vi "GUI FOFB Configuration Window.vi"(9 "username":string, 10 "password":string, 11 "FOFB-Controller IP Address in":string="10.0.5.31") -> (3 "Cancelled?":bool)   [LabVIEW 2011, in "User Interface Window VIs.lvlib"]
doc: "Fast Orbit Feedback (FOFB) graphical user interface."
uses:
  User Interface Window VIs.lvlib
  Types Definitions/Type BPM or PS Selector.ctl
  Types Definitions/Type FOFB Parameters.ctl
  Types Definitions/Type Network Configuration.ctl
  Types Definitions/Type FA Configuration.ctl
  Types Definitions/Type Response Matrix Measurement Configuration.ctl
  Types Definitions/Type Correction Algorithm Configuration.ctl
  Types Definitions/Type Acquisition Network Configuration.ctl
  Types Definitions/Type Actuation Network Configuration.ctl
  Types Definitions/Type FOFB GUI.ctl
  Types Definitions/Type Configuration Loop Mode.ctl
  Types Definitions/Type Configuration Data (GUI to Controller).ctl
  Types Definitions/Type Monitoring Data.ctl
  Types Definitions/Type Diagnostics Data.ctl
  Types Definitions/Type CPU Loads Array.ctl
  Types Definitions/Type CPU Loads.ctl
  Types Definitions/Type Diagnostics Sample.ctl
  Types Definitions/Type Monitoring Sample.ctl
  User Interface VIs.lvlib
  Type Definitions.lvlib
  XML VIs.lvlib
panel:
  in  "FOFB GUI In":T1
  out "FOFB Parameters Out":T2
  in  "FOFB Parameters In":T2
  in  "Refresh Button":bool
  out "Response Matrix List":string[](array[string]) caption="Lista de Matrizes Resposta"
  in  "Response Matrix":string caption="Matriz Resposta Escolhida"
  in  "PS Group ALV":bool
  in  "PS Group ACV":bool
  in  "PS Group ACH":bool
  in  "BPM Selector Vertical":bool
  in  "BPM Selector Horizontal":bool
  in  "PS Graph Selector ALV":T9[](array[typedef]) caption="Grupo ALV"
  in  "PS Graph Selector Vertical":T9[](array[typedef]) caption="Grupo ACV"
  in  "PS Graph Selector Horizontal":T9[](array[typedef]) caption="Grupo ACH"
  in  "BPM Graph Selector Vertical":T9[](array[typedef]) caption="BPMs Verticais"
  in  "BPM Graph Selector Horizontal":T9[](array[typedef]) caption="BPMs Horizontais"
  in  "Cancel Button":bool
  in  "OK Button":bool
  in  "BPM Graph Selector":T9[](array[typedef]) caption="BPMs"
  in  "Vertical (%)":dbl
  in  "Horizontal (%)":dbl
  # "Todos/Nenhum"
  # "Todos/Nenhum"
  # "Todos/Nenhum"
  # "Todos/Nenhum"
  # "Todos/Nenhum"
  # "Fator de correção"
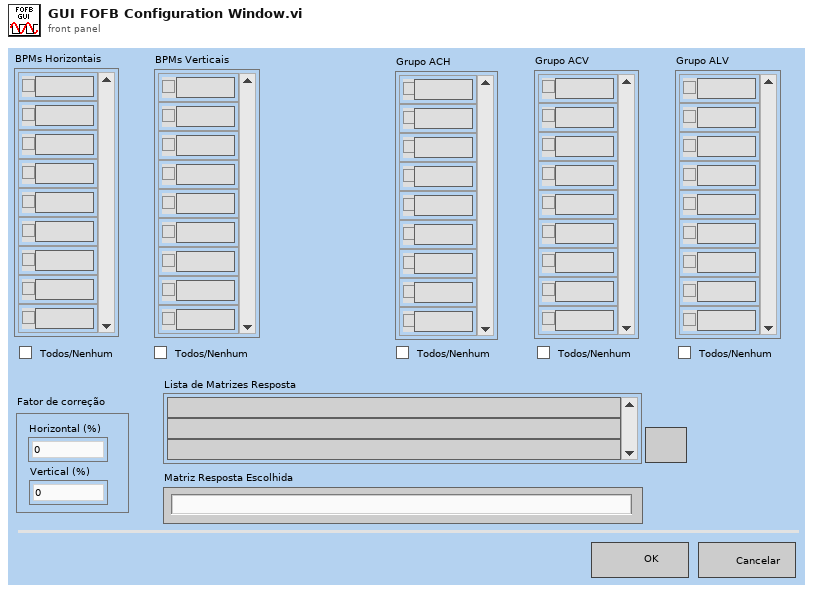
[diagram p1: front panel]
types:
  T1 = typedef "Type Definitions.lvlib/Type FOFB GUI.ctl" = cluster{"Response Matrix List Folder Notifier":refnum<notifier>, "Send Reference Orbit Notifier":refnum<notifier>, "FOFB Parameters Notifier":refnum<notifier>, "Configuration Loop Mode Notifier":refnum<notifier>, "Stop VIs Notifier":refnum<notifier>, "GUI Configuration Notifier":refnum<notifier>, "Monitoring Data Notifier":refnum<queue>, "Performance Monitoring Data Notifier":refnum<queue>, "BPM / PS Monitoring Data Notifiers":refnum<queue>[], "Load Orbit Notifier":refnum<notifier>, "RMS Monitoring Data Queue":refnum<queue>, "GUI-Controller Connected Queue":refnum<queue>}
  T2 = typedef "Type Definitions.lvlib/Type FOFB Parameters.ctl" = cluster{"Network":T3, "Fast Acquisition":T4, "Response Matrix Measurement":T5, "Correction Algorithm":T6, "Acquisition Network":T7, "Actuation Network":T8}
  T3 = typedef "Type Definitions.lvlib/Type Network Configuration.ctl" = cluster{"FOFB Controller IP":string, "LNLS Control Network IP":string, "LNLS Control Network Power Supplies TCP Port":u16, "LNLS Control Network FOFB Configuration TCP Port":u16, "Data Server TCP Port":u16, "Monitoring Data TCP Port":u16, "Configuration GUI TCP Port":u16, "TCP Listening Timeout":i32}
  T4 = typedef "Type Definitions.lvlib/Type FA Configuration.ctl" = cluster{"Acquisition Period":u32, "Data Buffer Size":u32, "Monitoring Period":u32}
  T5 = typedef "Type Definitions.lvlib/Type Response Matrix Measurement Configuration.ctl" = cluster{"Step Amplitude":dbl, "Time Between Steps":u32, "Step Duration":u32, "Number of Averages":u32}
  T6 = typedef "Type Definitions.lvlib/Type Correction Algorithm Configuration.ctl" = cluster{"Correction Period":u32, "Reference Orbit Path":path, "Response Matrix Path":path, "Correction Matrix Path":path, "Horizontal Correction Factor":dbl, "Vertical Correction Factor":dbl, "Beam Current FOFB Threshold":dbl, "Decouple H-V":bool, "Use Additional BPM LPF":bool, "BPM LPF Cutoff":dbl}
  T7 = typedef "Type Definitions.lvlib/Type Acquisition Network Configuration.ctl" = cluster{"Chassis Name":string, "Variables":cluster{"Variable Name":string, "Matrix Order":u32, "Location":dbl, "Plane":enum8{"H", "V"}, "On Correction":bool}[]}[]
  T8 = typedef "Type Definitions.lvlib/Type Actuation Network Configuration.ctl" = cluster{"Chassis Name":string, "Variables":cluster{"Variable Name":string, "Matrix Order":u32, "RMM Step Factor":dbl, "Plane":enum8{"H", "V"}, "On Correction":bool, "Kc":dbl, "Ti":dbl, "Td":dbl}[]}[]
  T9 = typedef "Type Definitions.lvlib/Type BPM or PS Selector.ctl" = cluster{"Name":string, "Active":bool}
  T10 = typedef "Type Definitions.lvlib/Type Configuration Loop Mode.ctl" = enum8{"Operation Mode", "Request FOFB Parameters", "Send New FOFB Parameters", "Send Reference Orbit", "Request Response Matrix List Folder"}
  T11 = typedef "Type Definitions.lvlib/Type PS Parameters.ctl" = cluster{"RMM Step Factor":dbl, "Plane":enum8{"H", "V"}, "On Correction":bool}
  T12 = typedef "Type Definitions.lvlib/Type BPM Parameters.ctl" = cluster{"Location":dbl, "Plane":enum8{"H", "V"}, "On Correction":bool}
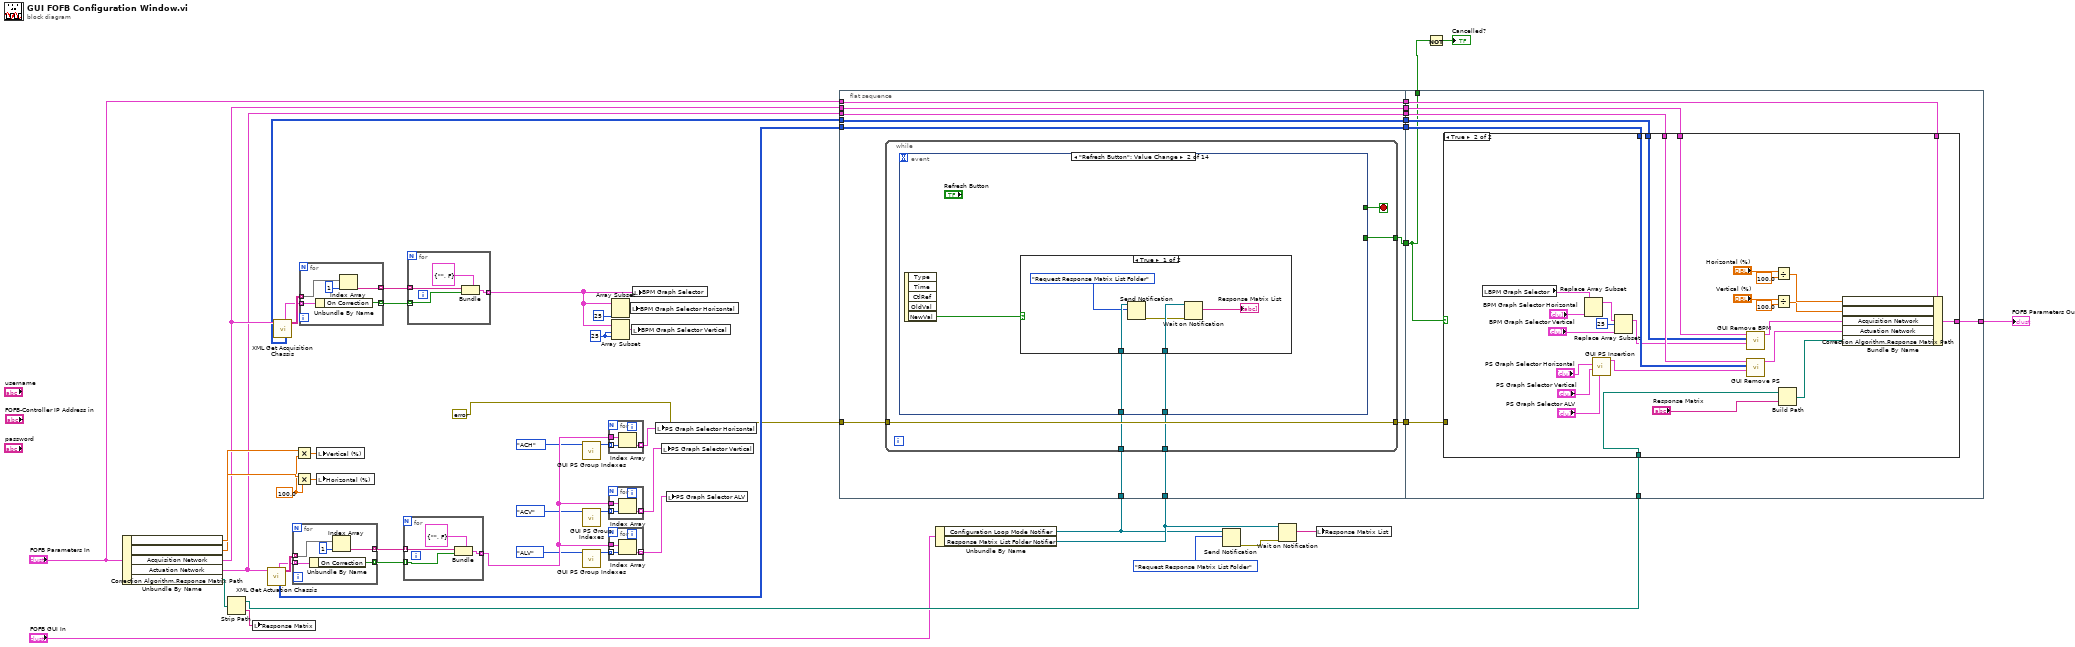
[diagram p0: block diagram]
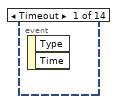
[diagram p2: hidden frame]
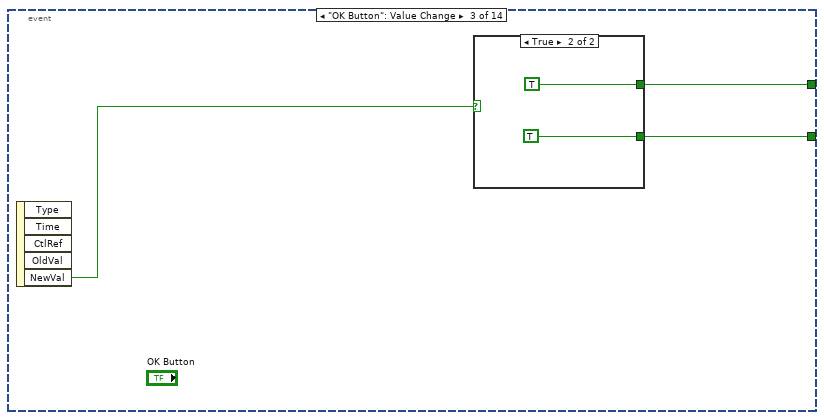
[diagram p4: hidden frame]
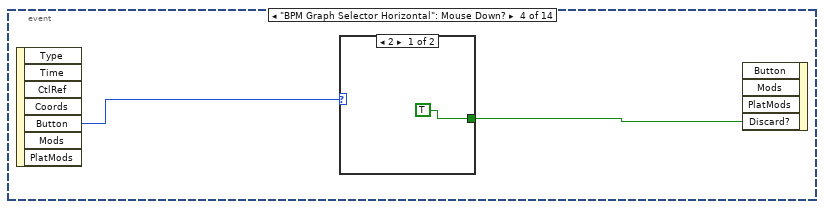
[diagram p6: hidden frame]
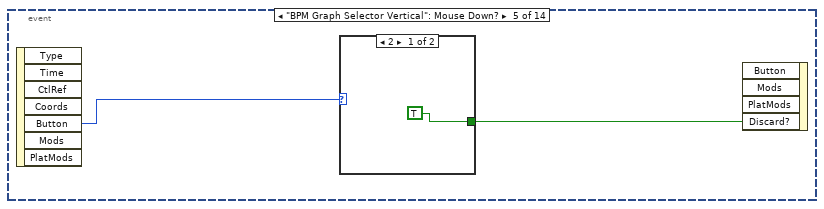
[diagram p8: hidden frame]
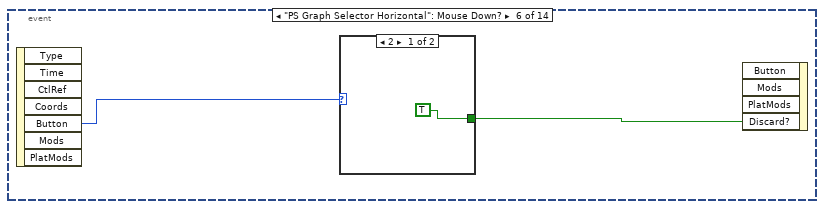
[diagram p10: hidden frame]
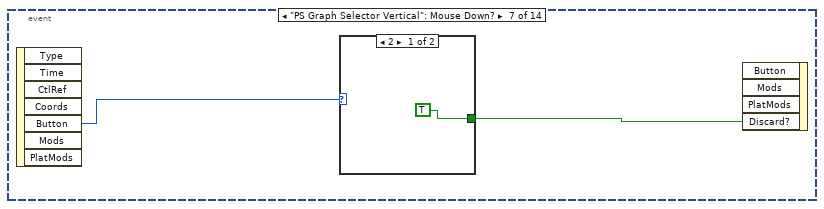
[diagram p12: hidden frame]
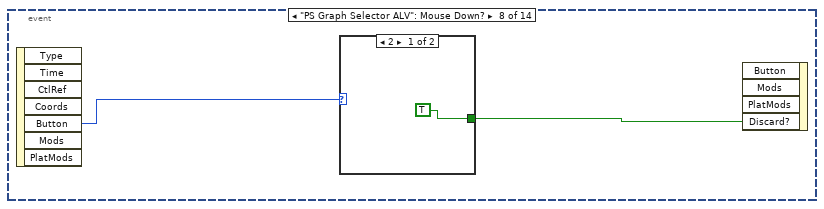
[diagram p14: hidden frame]
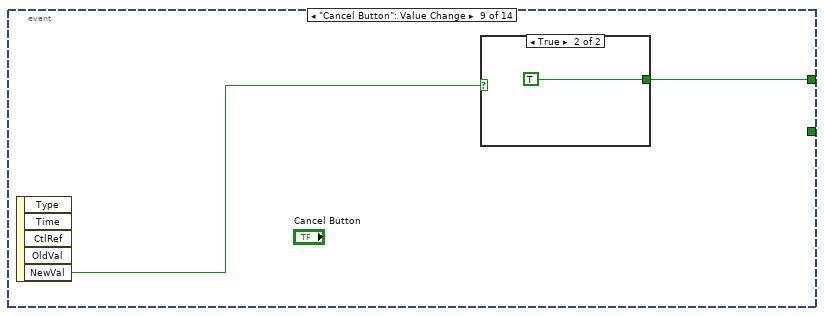
[diagram p16: hidden frame]
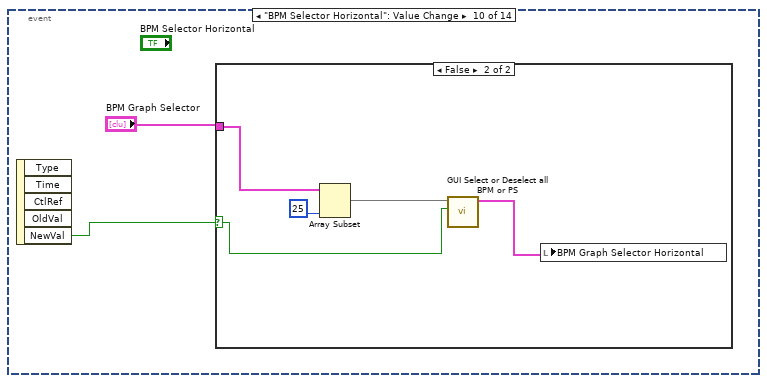
[diagram p18: hidden frame]
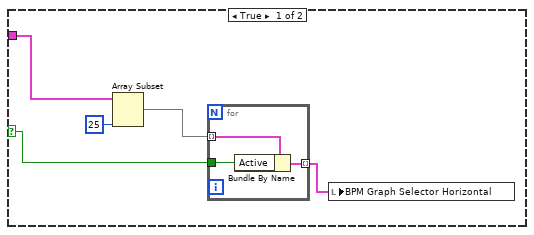
[diagram p19: hidden frame]
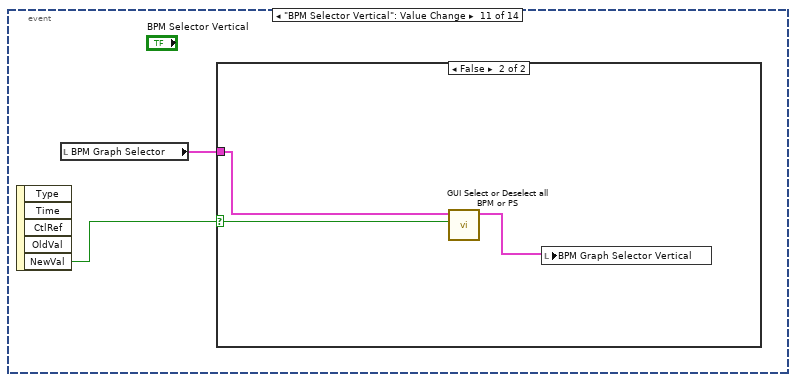
[diagram p20: hidden frame]
diagram:
  w17 = 25 ("index")
  w40 = 100.0 ("y")
  n1 = Unbundle By Name("FOFB Parameters In") -> ("Correction Algorithm.Horizontal Correction Factor"=w43:dbl, "Correction Algorithm.Vertical Correction Factor"=w42:dbl, "Acquisition Network"=w39:T7, "Actuation Network"=w38:T8, "Correction Algorithm.Response Matrix Path"=w31:path)
  n2 = Strip Path(path=w31) -> (stripped path=w30:path, name=w32:string)
  n3 = local write "Response Matrix"(w32) -> ()
  n4 = call "XML Get Actuation Chassis.vi"("Actuation Network"=w38) -> ("Actuation Variable Names"=w49:string[][], "Inverse PS Matrix Mapping"=w36:u32[][], "PS Parameters"=w48:T11[])  [unwired: 3 in, 5 out]
  n5 = call "XML Get Acquisition Chassis.vi"("Acquisition Network"=w39) -> ("Acquisition Variable Names"=w52:string[][], "Inverse BPM Matrix Mapping"=w37:u32[][], "BPM Parameters"=w47:T12[])  [unwired: 4 in, 4 out]
  n6 = for {
    tunnel: w49 -> [w57] mode=indexing
    tunnel: [w56] -> w46 mode=indexing
    tunnel: w48 -> [w55] mode=indexing
    tunnel: [w54] -> w45 mode=indexing
    n7 = Unbundle By Name(w55) -> ("On Correction"=w54:bool)
    n8 = Index Array(array=w57, index=1) -> (element=w56:string)
  }
  n9 = Multiply(x=w42, y=w40) -> (x*y=w41:dbl)
  n10 = Multiply(x=w43, y=w40) -> (x*y=w44:dbl)
  n11 = for {
    tunnel: w52 -> [w62] mode=indexing
    tunnel: [w61] -> w50 mode=indexing
    tunnel: w47 -> [w60] mode=indexing
    tunnel: [w59] -> w51 mode=indexing
    n12 = Unbundle By Name(w60) -> ("On Correction"=w59:bool)
    n13 = Index Array(array=w62, index=1) -> (element=w61:string)
  }
  n14 = local write "Vertical (%)"(w41) -> ()
  n15 = local write "Horizontal (%)"(w44) -> ()
  n16 = for {
    tunnel: [w66] -> w33 mode=indexing
    tunnel: w45 -> [w64] mode=indexing
    tunnel: w46 -> [w65] mode=indexing
    n17 = Bundle(cluster=T9 {"Name"="", "Active"=FALSE} ("BPM or PS Selection"), "Name"=w65, "Active"=w64) -> (w66:T9)
  }
  n18 = for {
    tunnel: [w70] -> w34 mode=indexing
    tunnel: w51 -> [w68] mode=indexing
    tunnel: w50 -> [w69] mode=indexing
    n19 = Bundle(cluster=T9 {"Name"="", "Active"=FALSE} ("BPM or PS Selection"), "Name"=w69, "Active"=w68) -> (w70:T9)
  }
  n20 = call "GUI PS Group Indexes.vi"("PS Group"=enum16{"ACH", "ACV", "ALV"}."ACH") -> ("Indexes"=w13:i32[])  [unwired: 10 in]
  n21 = call "GUI PS Group Indexes.vi"("PS Group"=enum16{"ACH", "ACV", "ALV"}."ACV") -> ("Indexes"=w11:i32[])  [unwired: 10 in]
  n22 = call "GUI PS Group Indexes.vi"("PS Group"=enum16{"ACH", "ACV", "ALV"}."ALV") -> ("Indexes"=w10:i32[])  [unwired: 10 in]
  n23 = for {
    tunnel: w33 -> [w74]
    tunnel: [w73] -> w15 mode=indexing
    tunnel: w13 -> [w72] mode=indexing
    n24 = Index Array(array=w74, index=w72) -> (element=w73:T9)
  }
  n25 = for {
    tunnel: w33 -> [w77]
    tunnel: [w76] -> w12 mode=indexing
    tunnel: w11 -> [w75] mode=indexing
    n26 = Index Array(array=w77, index=w75) -> (element=w76:T9)
  }
  n27 = for {
    tunnel: w33 -> [w80]
    tunnel: [w79] -> w14 mode=indexing
    tunnel: w10 -> [w78] mode=indexing
    n28 = Index Array(array=w80, index=w78) -> (element=w79:T9)
  }
  n29 = Array Subset(array=w34, length=25) -> (w18:T9[])  [unwired: 1 in]
  n30 = Array Subset(array=w34, index=w17, length=w17) -> (w19:T9[])
  n31 = local write "BPM Graph Selector Horizontal"(w18) -> ()
  n32 = local write "BPM Graph Selector Vertical"(w19) -> ()
  n33 = local write "BPM Graph Selector"(w34) -> ()
  n34 = local write "PS Graph Selector Horizontal"(w15) -> ()
  n35 = local write "PS Graph Selector Vertical"(w12) -> ()
  n36 = local write "PS Graph Selector ALV"(w14) -> ()
  n37 = flat-sequence {
    tunnel: errorcluster {"status"=FALSE, "code"=0, "source"=""} ("error in (no error)") -> [w83]
    tunnel: "FOFB Parameters In" -> [w89]
    tunnel: w39 -> [w88]
    tunnel: w38 -> [w87]
    tunnel: w37 -> [w86]
    tunnel: w36 -> [w85]
    tunnel: [w90] -> w26
    tunnel: [w89] -> w25
    tunnel: [w88] -> w24
    tunnel: [w87] -> w23
    tunnel: [w86] -> w22
    tunnel: [w85] -> w21
    tunnel: [w84] -> w20
    tunnel: w2 -> [w82]
    tunnel: w3 -> [w81]
    tunnel: w26 -> [w187]
    tunnel: w25 -> [w194]
    tunnel: w24 -> [w193]
    tunnel: w23 -> [w192]
    tunnel: w22 -> [w191]
    tunnel: w21 -> [w190]
    tunnel: [w187] -> w35
    tunnel: w30 -> [w189]
    tunnel: w20 -> [w188]
    tunnel: [w186] -> w27
    frame #0 {
      n38 = while {
        tunnel: w83 -> [w95]
        tunnel: [w95] -> w84
        tunnel: [w93] -> w90
        tunnel: w82 -> [w92]
        tunnel: w81 -> [w91]
        stop <- w94 stop-if-true
        n39 = event shown="[1] \"Refresh Button\": Value Change" {
          selector: _ -> [_ _ _ _ _ _ _ _ _ _ _ _ _ _]
          dyn-events: _ -> [_ _ _ _ _ _ _ _ _ _ _ _ _ _]
          timeout: _ -> [_ _ _ _ _ _ _ _ _ _ _ _ _ _]
          tunnel: [_ _ w106 _ _ _ _ _ w125 _ _ _ _ _] -> w94
          tunnel: [_ _ w105 _ _ _ _ _ _ _ _ _ _ _] -> w93
          tunnel: w92 -> [_ w97 _ _ _ _ _ _ _ _ _ _ _ _]
          tunnel: w91 -> [_ w96 _ _ _ _ _ _ _ _ _ _ _ _]
          event Timeout {
            n40 = event-data() -> ()  [unwired: 1 in, 2 out]
          }
          event "Refresh Button": Value Change {
            n41 = event-data() -> ("NewVal"=w98:bool)  [unwired: 1 in, 4 out]
            n42 = case shown="True" w98 {
              tunnel: w97 -> [w103 _]
              tunnel: w96 -> [w102 _]
              frame True {
                n43 = Send Notification(notification=Type_Configuration_Loop_Mode."Request Response Matrix List Folder", notifier=w103) -> (error out=w100:errorcluster)  [unwired: 1 in, 1 out]
                n44 = Wait on Notification(notifier=w102, error in (no error)=w100) -> (notification=→"Response Matrix List":string[])  [unwired: 2 in, 3 out]
              }
              frame False {
              }
            }
          }
          event "OK Button": Value Change {
            n45 = event-data() -> ("NewVal"=w104:bool)  [unwired: 1 in, 4 out]
            n46 = case shown="True" w104 {
              tunnel: [_ TRUE] -> w106
              tunnel: [_ TRUE] -> w105
              frame False {
              }
              frame True {
              }
            }
          }
          event "BPM Graph Selector Horizontal": Mouse Down? {
            n47 = event-data() -> ("Button"=w110:u16)  [unwired: 1 in, 6 out]
            n48 = case shown="2" w110 {
              tunnel: [TRUE ("Discard?") _] -> w109
              frame 2 {
              }
              frame 1, Default {
              }
            }
            n49 = event-data("Discard?"=w109) -> ()  [unwired: 4 in, 1 out]
          }
          event "BPM Graph Selector Vertical": Mouse Down? {
            n50 = event-data() -> ("Button"=w113:u16)  [unwired: 1 in, 6 out]
            n51 = case shown="2" w113 {
              tunnel: [TRUE ("Discard?") _] -> w112
              frame 2 {
              }
              frame 1, Default {
              }
            }
            n52 = event-data("Discard?"=w112) -> ()  [unwired: 4 in, 1 out]
          }
          event "PS Graph Selector Horizontal": Mouse Down? {
            n53 = event-data() -> ("Button"=w116:u16)  [unwired: 1 in, 6 out]
            n54 = case shown="2" w116 {
              tunnel: [TRUE ("Discard?") _] -> w115
              frame 2 {
              }
              frame 1, Default {
              }
            }
            n55 = event-data("Discard?"=w115) -> ()  [unwired: 4 in, 1 out]
          }
          event "PS Graph Selector Vertical": Mouse Down? {
            n56 = event-data() -> ("Button"=w119:u16)  [unwired: 1 in, 6 out]
            n57 = case shown="2" w119 {
              tunnel: [TRUE ("Discard?") _] -> w118
              frame 2 {
              }
              frame 1, Default {
              }
            }
            n58 = event-data("Discard?"=w118) -> ()  [unwired: 4 in, 1 out]
          }
          event "PS Graph Selector ALV": Mouse Down? {
            n59 = event-data() -> ("Button"=w122:u16)  [unwired: 1 in, 6 out]
            n60 = case shown="2" w122 {
              tunnel: [TRUE ("Discard?") _] -> w121
              frame 2 {
              }
              frame 1, Default {
              }
            }
            n61 = event-data("Discard?"=w121) -> ()  [unwired: 4 in, 1 out]
          }
          event "Cancel Button": Value Change {
            n62 = event-data() -> ("NewVal"=w124:bool)  [unwired: 1 in, 4 out]
            n63 = case shown="True" w124 {
              tunnel: [_ TRUE] -> w125
              frame False {
              }
              frame True {
              }
            }
          }
          event "BPM Selector Horizontal": Value Change {
            n64 = event-data() -> ("NewVal"=w128:bool)  [unwired: 1 in, 4 out]
            n65 = case shown="False" w128 {
              selector: w128 -> [w131 w137]
              tunnel: "BPM Graph Selector" -> [w129 w140]
              frame True {
                n66 = Array Subset(array=w129, length=25) -> (w132:T9[])  [unwired: 1 in]
                n67 = for {
                  tunnel: w132 -> [w135] mode=indexing
                  tunnel: [w136] -> w130 mode=indexing
                  tunnel: w131 -> [w134]
                  n68 = Bundle By Name(cluster=w135, "Active"=w134) -> (w136:T9)
                }
                n69 = local write "BPM Graph Selector Horizontal"(w130) -> ()
              }
              frame False {
                n70 = Array Subset(array=w140, length=25) -> (w139:T9[])  [unwired: 1 in]
                n71 = call "GUI Select or Deselect all BPM or PS.vi"("Boolean Value"=w137, "Variable Selector In"=w139) -> ("Variable Selector Out"=w138:T9[])  [unwired: 8 in, 1 out]
                n72 = local write "BPM Graph Selector Horizontal"(w138) -> ()
              }
            }
          }
          event "BPM Selector Vertical": Value Change {
            n73 = event-data() -> ("NewVal"=w143:bool)  [unwired: 1 in, 4 out]
            n74 = local read "BPM Graph Selector"() -> (w142:T9[])
            n75 = case shown="False" w143 {
              selector: w143 -> [w146 w151]
              tunnel: w142 -> [w144 w152]
              frame True {
                n76 = for {
                  tunnel: w144 -> [w148] mode=indexing
                  tunnel: [w149] -> w145 mode=indexing
                  tunnel: w146 -> [w147]
                  n77 = Bundle By Name(cluster=w148, "Active"=w147) -> (w149:T9)
                }
                n78 = local write "BPM Graph Selector Vertical"(w145) -> ()
              }
              frame False {
                n79 = call "GUI Select or Deselect all BPM or PS.vi"("Boolean Value"=w151, "Variable Selector In"=w152) -> ("Variable Selector Out"=w150:T9[])  [unwired: 8 in, 1 out]
                n80 = local write "BPM Graph Selector Vertical"(w150) -> ()
              }
            }
          }
          event "PS Group ACH": Value Change {
            n81 = event-data() -> ("NewVal"=w154:bool)  [unwired: 1 in, 4 out]
            n82 = local read "PS Graph Selector Horizontal"() -> (w153:T9[])
            n83 = case shown="True" w154 {
              selector: w154 -> [w155 w160]
              tunnel: w153 -> [w157 w158]
              frame True {
                n84 = call "GUI Select or Deselect all BPM or PS.vi"("Boolean Value"=w155, "Variable Selector In"=w157) -> ("Variable Selector Out"=w156:T9[])  [unwired: 8 in, 1 out]
                n85 = local write "PS Graph Selector Horizontal"(w156) -> ()
              }
              frame False {
                n86 = for {
                  tunnel: w158 -> [w163] mode=indexing
                  tunnel: [w162] -> w159 mode=indexing
                  tunnel: w160 -> [w161]
                  n87 = Bundle By Name(cluster=w163, "Active"=w161) -> (w162:T9)
                }
                n88 = local write "PS Graph Selector Horizontal"(w159) -> ()
              }
            }
          }
          event "PS Group ACV": Value Change {
            n89 = local read "PS Graph Selector Vertical"() -> (w164:T9[])
            n90 = event-data() -> ("NewVal"=w165:bool)  [unwired: 1 in, 4 out]
            n91 = case shown="True" w165 {
              selector: w165 -> [w166 w171]
              tunnel: w164 -> [w168 w169]
              frame True {
                n92 = call "GUI Select or Deselect all BPM or PS.vi"("Boolean Value"=w166, "Variable Selector In"=w168) -> ("Variable Selector Out"=w167:T9[])  [unwired: 8 in, 1 out]
                n93 = local write "PS Graph Selector Vertical"(w167) -> ()
              }
              frame False {
                n94 = for {
                  tunnel: w169 -> [w174] mode=indexing
                  tunnel: [w173] -> w170 mode=indexing
                  tunnel: w171 -> [w172]
                  n95 = Bundle By Name(cluster=w174, "Active"=w172) -> (w173:T9)
                }
                n96 = local write "PS Graph Selector Vertical"(w170) -> ()
              }
            }
          }
          event "PS Group ALV": Value Change {
            n97 = event-data() -> ("NewVal"=w176:bool)  [unwired: 1 in, 4 out]
            n98 = local read "PS Graph Selector ALV"() -> (w175:T9[])
            n99 = case shown="False" w176 {
              selector: w176 -> [w177 w182]
              tunnel: w175 -> [w179 w180]
              frame False {
                n100 = call "GUI Select or Deselect all BPM or PS.vi"("Boolean Value"=w177, "Variable Selector In"=w179) -> ("Variable Selector Out"=w178:T9[])  [unwired: 8 in, 1 out]
                n101 = local write "PS Graph Selector ALV"(w178) -> ()
              }
              frame True {
                n102 = for {
                  tunnel: w180 -> [w185] mode=indexing
                  tunnel: [w184] -> w181 mode=indexing
                  tunnel: w182 -> [w183]
                  n103 = Bundle By Name(cluster=w185, "Active"=w183) -> (w184:T9)
                }
                n104 = local write "PS Graph Selector ALV"(w181) -> ()
              }
            }
          }
        }
      }
    }
    frame #1 {
      n105 = case shown="True" w187 {
        tunnel: w194 -> [_ w221]
        tunnel: w193 -> [_ w220]
        tunnel: w192 -> [_ w219]
        tunnel: w191 -> [_ w218]
        tunnel: w190 -> [_ w217]
        tunnel: w189 -> [_ w216]
        tunnel: w188 -> [_ _]
        tunnel: [_ w195] -> w186
        frame False {
        }
        frame True {
          n106 = local read "BPM Graph Selector"() -> (w211:T9[])
          n107 = Replace Array Subset(array=w211, new element="BPM Graph Selector Horizontal") -> (w214:T9[])  [unwired: 1 in]
          n108 = call "GUI PS Insertion.vi"("PS Graph Selector ALV"="PS Graph Selector ALV", "PS Graph Selector Vertical"="PS Graph Selector Vertical", "PS Graph Selector Horizontal"="PS Graph Selector Horizontal") -> ("PS Graph Selector out"=w208:T9[])  [unwired: 8 in]
          n109 = Replace Array Subset(array=w214, new element="BPM Graph Selector Vertical", index=25) -> (w210:T9[])
          n110 = call "GUI Remove BPM.vi"("BPM Graph Selector"=w210, "Inverse BPM Matrix Mapping"=w218, "Acquisition Network in"=w220) -> ("Acquisition Network out"=w203:T7)  [unwired: 8 in]
          n111 = call "GUI Remove PS.vi"("PS Graph Selector"=w208, "Inverse PS Matrix Mapping"=w217, "Actuation Network in"=w219) -> ("Actuation Network out"=w202:T8)  [unwired: 8 in]
          n112 = Divide(x="Horizontal (%)", y=100.0) -> (x/y=w199:dbl)
          n113 = Divide(x="Vertical (%)", y=100.0) -> (x/y=w198:dbl)
          n114 = Build Path(base path=w216, name or relative path="Response Matrix") -> (appended path=w197:path)
          n115 = Bundle By Name(cluster=w221, "Correction Algorithm.Horizontal Correction Factor"=w199, "Correction Algorithm.Vertical Correction Factor"=w198, "Acquisition Network"=w203, "Actuation Network"=w202, "Correction Algorithm.Response Matrix Path"=w197) -> (w195:T2)
        }
      }
    }
  }
  n116 = Unbundle By Name("FOFB GUI In") -> ("Configuration Loop Mode Notifier"=w2:refnum<notifier>, "Response Matrix List Folder Notifier"=w3:refnum<notifier>)
  n117 = Send Notification(notification=Type_Configuration_Loop_Mode."Request Response Matrix List Folder", notifier=w2) -> (error out=w5:errorcluster)  [unwired: 1 in, 1 out]
  n118 = Wait on Notification(notifier=w3, error in (no error)=w5) -> (notification=w1:string[])  [unwired: 2 in, 3 out]
  n119 = local write "Response Matrix List"(w1) -> ()
  n120 = Not(x=w35) -> (.not. x?=→"Cancelled?":bool)
  "FOFB Parameters Out" <- w27
